vi "List_Data_Files.vi"(7 "Drifter":i32, 8 "Error In":errorcluster, 11 "Drfiter IP Addresses":string[][](array[string])) -> (0 "Error Out":errorcluster, 2 "File List Array":string[](array[string]), 3 "File List":string)   [LabVIEW 2017]
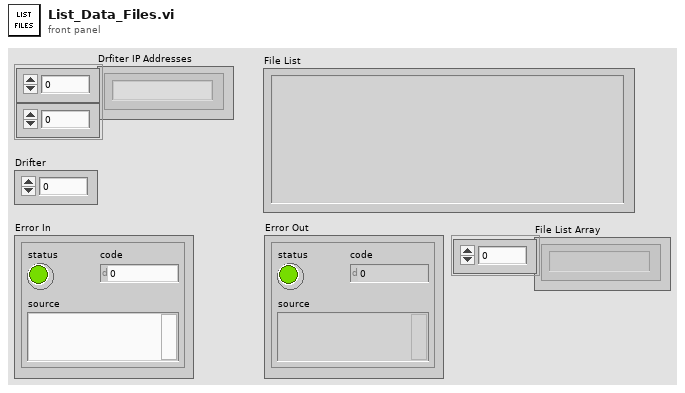
[diagram p1: front panel]
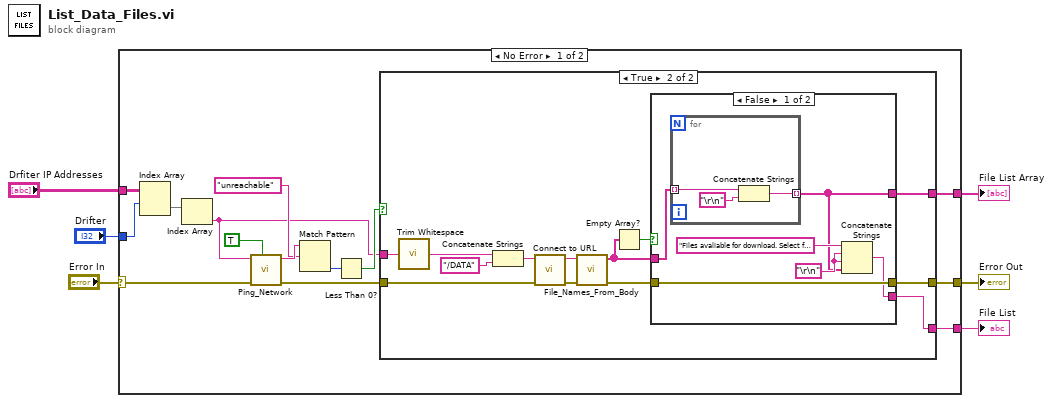
[diagram p0: block diagram]
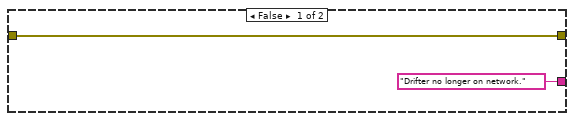
[diagram p2: hidden frame]
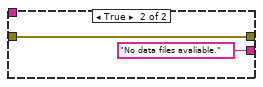
[diagram p3: hidden frame]
diagram:
  n1 = case shown="No Error" "Error In" {
    selector: "Error In" -> [w7 w47]
    tunnel: [w20 w47] -> w6
    tunnel: "Drifter" -> [w19 _]
    tunnel: "Drfiter IP Addresses" -> [w11 _]
    tunnel: [w9 _] -> w3
    tunnel: [w8 _] -> w2
    frame No Error {
      n2 = Index Array(array=w11, index (row)=w19) -> (element=w18:string[])  [unwired: 1 in]
      n3 = Index Array(array=w18) -> (element=w10:string)  [unwired: 1 in]
      n4 = call "Ping_Network.vi"("IP/Default Gateway (T/F)"=TRUE, "Error In"=w7, "Default Gateway/IP"=w10) -> ("Error Out"=w12:errorcluster, "Terminal Output"=w16:string)  [unwired: 7 in]
      n5 = Match Pattern(string=w16, regular expression="unreachable") -> (offset past match=w14:i32)  [unwired: 1 in, 3 out]
      n6 = Less Than 0?(x=w14) -> (x < 0?=w13:bool)
      n7 = case shown="True" w13 {
        tunnel: w12 -> [w22 w35]
        tunnel: [w22 w24] -> w20
        tunnel: w10 -> [_ w31]
        tunnel: ["Drifter no longer on network." ("Body") w27] -> w9
        tunnel: [_ w23] -> w8
        frame False {
        }
        frame True {
          n8 = call <vilib>:"Trim Whitespace.vi"("string"=w31) -> ("trimmed string"=w34:string)  [unwired: 1 in]
          n9 = Concatenate Strings(w34, "/DATA" ("string")) -> (w32:string)
          n10 = call "Connect to URL.vi"("Error In"=w35, "URL"=w32) -> ("Error Out"=w29:errorcluster, "Body"=w30:string)  [unwired: 8 in]
          n11 = call "File_Names_From_Body.vi"("Error In"=w29, "Body"=w30) -> ("Error OUt"=w25:errorcluster, "File Names"=w26:string[])  [unwired: 8 in]
          n12 = Empty Array?(array=w26) -> (empty?=w28:bool)
          n13 = case shown="False" w28 {
            tunnel: [w38 "No data files avaliable." ("Body")] -> w27
            tunnel: w26 -> [w41 _]
            tunnel: w25 -> [w40 w45]
            tunnel: [w40 w45] -> w24
            tunnel: [w36 _] -> w23
            frame False {
              w37 = "\r\n"
              n14 = for {
                tunnel: w41 -> [w42] mode=indexing
                tunnel: [w43] -> w36 mode=indexing
                n15 = Concatenate Strings(w42, "\r\n") -> (w43:string)
              }
              n16 = Concatenate Strings("Files avaliable for download. Select file from drop-down meanu and click \"View File\" to view. Select \"Download\" to down the file or \"Download All\" to download all data from the current drifter.", w37, w37, w36) -> (w38:string)
            }
            frame True {
            }
          }
        }
      }
    }
    frame Error {
    }
  }
  "Error Out" <- w6
  "File List" <- w3
  "File List Array" <- w2
